vi "Obtain Default Broadcast Events.vi"(8 "error in":errorcluster) -> (0 "error out":errorcluster, 1 "Update Module Execution Status":refnum<user-event>, 2 "Error Reported":refnum<user-event>, 3 "Status Updated":refnum<user-event>, 4 "System Message":refnum<user-event>, 5 "Module Did Stop":refnum<user-event>)   [LabVIEW 2022 SP3, in "MainPanel.lvlib"]
doc: "Encapsulates the module-specific Obtain Broadcast Events for Registration.vi and only returns the default broadcast event references that any HSE DQMH module features. Wrapping the VI allows to programmatically obtain the default event references as the module-specific connector panes are hidden away. Event references returned are:\n\nStatus updated\nError reported\nModule Did Stop\nUpdate Module Execution Status\nSystem Message (HSE-specific event)"
uses:
  MainPanel.lvlib
  Status Updated Argument--cluster.ctl
  Error Reported Argument--cluster.ctl
  Stop Argument--cluster.ctl
  Get Module Execution Status Argument--cluster.ctl
  System Message Argument--cluster.ctl
  Libraries/hse-libraries/Source/hse-dqmh/Controls/System Message Source.ctl
  Libraries/hse-libraries/Source/hse-dqmh/hse-dqmh.lvlib
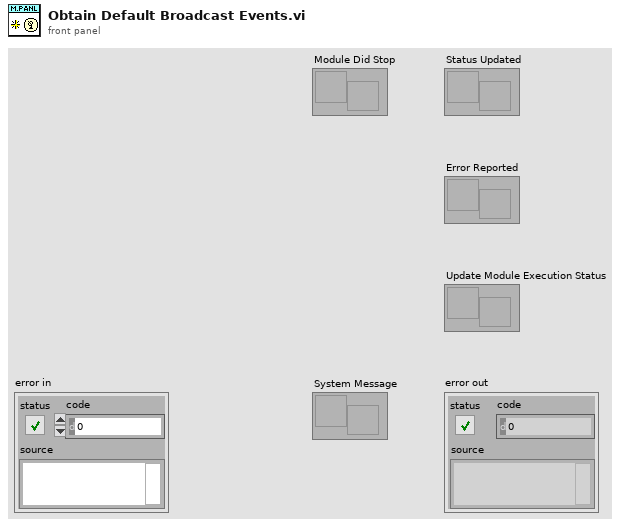
[diagram p1: front panel]
types:
  T1 = typedef "MainPanel.lvlib/Broadcast Events--cluster.ctl" = cluster{"Module Did Init":refnum<user-event>, "Status Updated":refnum<user-event>, "Error Reported":refnum<user-event>, "Did Something":refnum<user-event>, "Module Did Stop":refnum<user-event>, "Update Module Execution Status":refnum<user-event>, "System Message":refnum<user-event>}
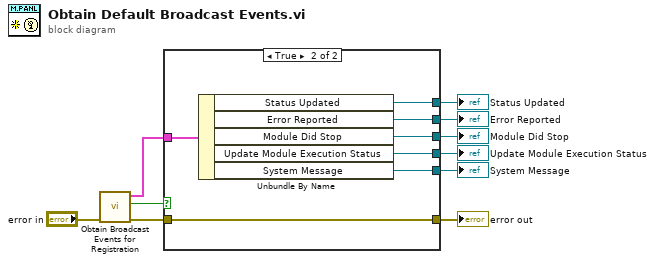
[diagram p0: block diagram]
diagram:
  n1 = call "Obtain Broadcast Events for Registration.vi"("error in"="error in") -> ("error out"=w9:errorcluster, "Already running?"=w1:bool, "MainPanel Broadcast Events"=w7:T1)  [unwired: 8 in]
  n2 = case shown="True" w1 {
    tunnel: w9 -> [w11 w18]
    tunnel: [w11 w18] -> w8
    tunnel: w7 -> [_ w17]
    tunnel: [_ w16] -> w6
    tunnel: [_ w15] -> w5
    tunnel: [_ w14] -> w4
    tunnel: [_ w13] -> w3
    tunnel: [_ w12] -> w2
    frame False {
    }
    frame True {
      n3 = Unbundle By Name(w17) -> ("Status Updated"=w16:refnum<user-event>, "Error Reported"=w15:refnum<user-event>, "Module Did Stop"=w14:refnum<user-event>, "Update Module Execution Status"=w13:refnum<user-event>, "System Message"=w12:refnum<user-event>)
    }
  }
  "error out" <- w8
  "Status Updated" <- w6
  "Error Reported" <- w5
  "Module Did Stop" <- w4
  "Update Module Execution Status" <- w3
  "System Message" <- w2
